vi "SaveAlmLog.vi"(8 "错误输入（无错误）":errorcluster, 11 "AlmLog":string) -> (0 "错误输出":errorcluster)   [LabVIEW 2017]
uses:
  Ctrls/PathChoose.ctl
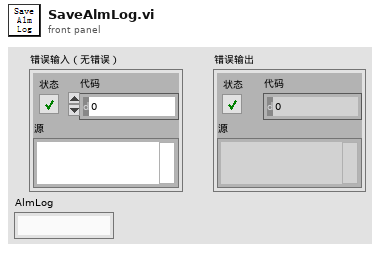
[diagram p1: front panel]
types:
  T1 = typedef "PathChoose.ctl" = enum16{"OperatorLog", "AutoRunLog", "AlmLog", "TestData", "AllTestData", "backup_nvm", "backup_before_flashing"}
  T2 = enum16{"open", "replace", "create", "open or create", "replace or create", "replace or create with confirmation"}
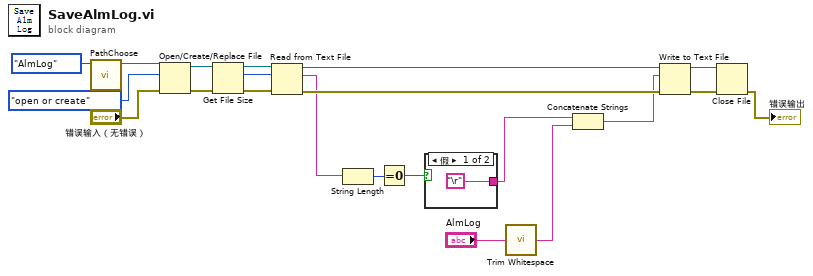
[diagram p0: block diagram]
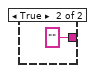
[diagram p2: hidden frame]
diagram:
  n1 = call "PathChoose.vi"(11:PathChoose."AlmLog") -> ("Path_Out"=w6:path)  [unwired: 10 in]
  n2 = Open/Create/Replace File(file path (use dialog)=w6, error in="错误输入（无错误）", operation (0:open)=T2."open or create" ("操作(0:open)")) -> (refnum out=w20:refnum<file>, error out=w19:errorcluster)  [unwired: 3 in, 1 out]
  n3 = Get File Size(file=w20, error in=w19) -> (refnum out=w18:refnum<file>, size (in bytes)=w16:i64, 0:w17:errorcluster)
  n4 = Read from Text File(file (use dialog)=w18, count=w16, error in=w17) -> (refnum out=w15:refnum<file>, text=w11:string, error out=w14:errorcluster)  [unwired: 1 in, 1 out]
  n5 = String Length(string=w11) -> (length=w12:i32)
  n6 = Equal To 0?(x=w12) -> (x = 0?=w13:bool)
  n7 = case shown="假" w13 {
    tunnel: ["\r" ""] -> w10
    frame False {
    }
    frame True {
    }
  }
  n8 = call <vilib>:"Trim Whitespace.vi"("string"="AlmLog") -> ("trimmed string"=w1:string)  [unwired: 1 in]
  n9 = Concatenate Strings(w10, w1) -> (w9:string)
  n10 = Write to Text File(file (use dialog)=w15, text=w9, error in=w14) -> (refnum out=w8:refnum<file>, error out=w7:errorcluster)  [unwired: 1 in, 1 out]
  n11 = Close File(refnum=w8, error in=w7) -> (error out=→"错误输出":errorcluster)  [unwired: 1 out]
